vi "AssetMgrDeviceDeletedBroadcast_Create.vi"(7 "Header":T2, 8 "error in (no error)":errorcluster, 11 "AssetMgrDeviceDeletedBroadcast":T1) -> (0 "error out":errorcluster, 3 "Message":T4)   [LabVIEW 2017]
uses:
  <vilib>/addons/InsightCM/MessageBus/Base/controls/Message.ctl
  <vilib>/addons/InsightCM/MessageBus/Base/controls/MessageHeader.ctl
  <vilib>/addons/InsightCM/MessageBus/Base/controls/KeyValuePair.ctl
  <vilib>/addons/InsightCM/MessageBus/MessageLibrary/AssetManager/controls/AssetMgrDeviceDeletedBroadcastBody.ctl
  <vilib>/addons/InsightCM/MessageBus/Base/controls/MessageClassType.ctl
  <vilib>/addons/InsightCM/Utilities/PropertyHelpers/PropertyHelpers.lvlib
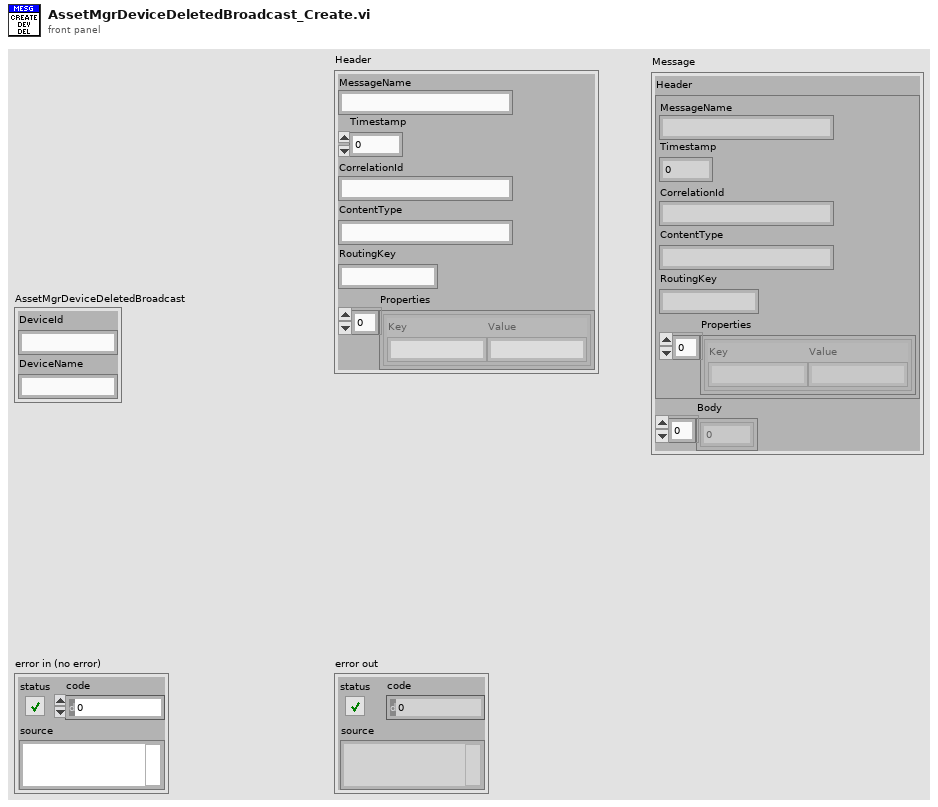
[diagram p1: front panel]
types:
  T1 = typedef "AssetMgrDeviceDeletedBroadcastBody.ctl" = cluster{"DeviceId":string, "DeviceName":string}
  T2 = typedef "MessageHeader.ctl" = cluster{"MessageName":string, "Timestamp":i64, "CorrelationId":string, "ContentType":string, "RoutingKey":string, "Properties":T3[]}
  T3 = typedef "KeyValuePair.ctl" = cluster{"Key":string, "Value":string}
  T4 = typedef "Message.ctl" = cluster{"Header":T2, "Body":u8[]}
  T5 = typedef "MessageClassType.ctl" = enum16{"Request", "Response", "Broadcast", "RoutedMessage"}
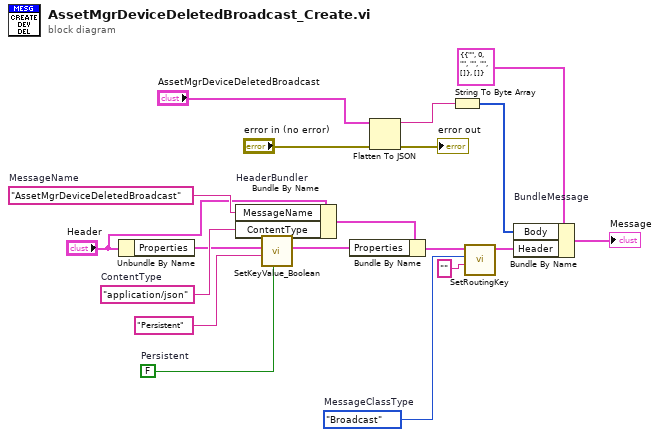
[diagram p0: block diagram]
diagram:
  w15 = MessageClassType."Broadcast"  # MessageClassType
  w10 = FALSE  # Persistent
  w16 = "AssetMgrDeviceDeletedBroadcast"  # MessageName
  w13 = "application/json"  # ContentType
  n1 = Unbundle By Name("Header") -> ("Properties"=w12:T3[])
  n2 = Bundle By Name "HeaderBundler"(cluster="Header", "MessageName"=w16, "ContentType"=w13) -> (w7:T2)
  n3 = call <vilib>:"SetKeyValue_Boolean.vi"("value"=w10, "key"="Persistent" ("Key"), "key value pairs"=w12) -> ("key value pairs out"=w6:T3[])  [unwired: 8 in]
  n4 = Bundle By Name(cluster=w7, "Properties"=w6) -> (w8:T2)
  n5 = Flatten To JSON(anything="AssetMgrDeviceDeletedBroadcast", error in (no error)="error in (no error)") -> (JSON string=w2:string, 11:→"error out":errorcluster)  [unwired: 1 in]
  n6 = String To Byte Array(string=w2) -> (unsigned byte array=w18:u8[])
  n7 = call <vilib>:"SetRoutingKey.vi"("SendTo"="", "MessageClassType"=w15, "Message Header in"=w8) -> ("Message Header out"=w9:T2)  [unwired: 8 in]
  n8 = Bundle By Name "BundleMessage"(cluster=T4 {"Header"={"MessageName"="", "Timestamp"=0, "CorrelationId"="", "ContentType"="", "RoutingKey"="", "Properties"=[]}, "Body"=[]} ("Message"), "Body"=w18, "Header"=w9) -> (→"Message":T4)
